vi "TempToVoltage.vi"(10 "T_out":dbl) -> (2 "u_out":dbl)   [LabVIEW 2019]
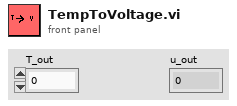
[diagram p1: front panel]
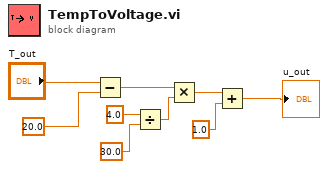
[diagram p0: block diagram]
diagram:
  n1 = Subtract(x="T_out", y=20.0) -> (x-y=w7:dbl)
  n2 = Divide(x=4.0, y=30.0) -> (x/y=w4:dbl)
  n3 = Multiply(x=w7, y=w4) -> (x*y=w3:dbl)
  n4 = Add(x=w3, y=1.0) -> (x+y=→"u_out":dbl)
